vi "Set LogEngine RawDataQs.vi"(8 "error in (no error)":errorcluster, 10 "LogEngine DataQs":T1, 11 "LogEngine.lvclass":refnum<class "LogEngine.lvclass">) -> (0 "error out":errorcluster, 3 "LogEngine.lvclass":refnum<class "LogEngine.lvclass">)   [LabVIEW 2017]
uses:
  LogEngine.lvclass
  DAQ/Process/ProcessSupport/TD local raw AI Data--cluster.ctl
  DAQ/DAQ.lvclass
  Data Types/TD Queues_LogEngine.ctl
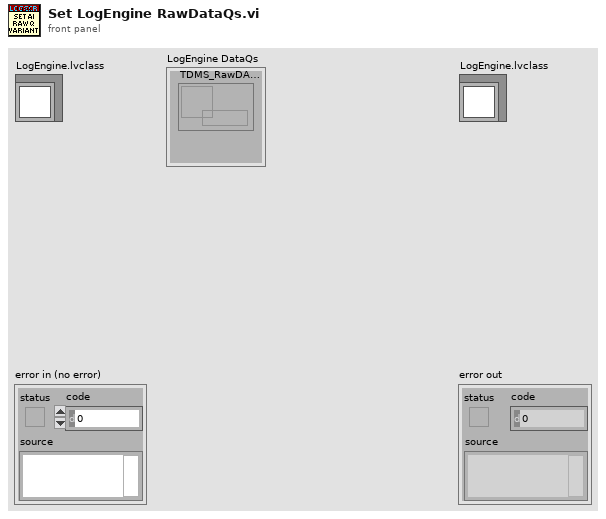
[diagram p1: front panel]
types:
  T1 = typedef "TD Queues_LogEngine.ctl" = cluster{"TDMS_RawDAQDataQ":refnum<queue>}
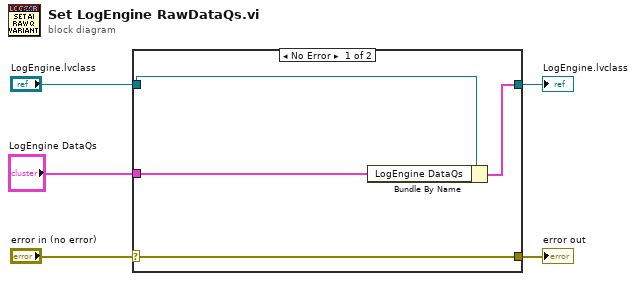
[diagram p0: block diagram]
diagram:
  n1 = case shown="No Error" "error in (no error)" {
    selector: "error in (no error)" -> [w9 w10]
    tunnel: [w9 w10] -> w4
    tunnel: [w7 w11] -> w2
    tunnel: "LogEngine.lvclass" -> [w8 w11]
    tunnel: "LogEngine DataQs" -> [w6 _]
    frame No Error {
      n2 = Bundle By Name(cluster=w8, "LogEngine DataQs"=w6) -> (w7:cluster{})
    }
    frame Error {
    }
  }
  "error out" <- w4
  "LogEngine.lvclass" <- w2
